vi "acquire data for calibration.vi"(0 "Connection ID":refnum<k5>, 7 "method":T2={"sampling interval"=0.1, "samples to average"=1, "data interval"=0.0, "stream data"=FALSE, "file path"=refnum, "command"={"command"=enum."Idle", "start time (ms)"=0, "Channel Indices"=[], "Scans per Sample"=1}} {"command"."Scans per Sample" min=1; "data interval" format="%.2f"; "samples to average" min=1 step=1; "sampling interval" format="%.2f"}, 9 "Reference Index":u32, 11 "Uncalibrated index":u32) -> (4 "data array":sgl[][](array[numeric]) format="%.5f", 6 "offset":sgl format="%.5f", 8 "percent CV":sgl format="%.5f")   [LabVIEW 2010]
uses:
  DataServer/Server Stats.vi
  DataServer/command.ctl
  DataServer/command cluster.ctl
  DAC apps/support/method.ctl
panel:
  in  "colors":i32[](array[numeric])=[16711680, 13311, 52224, 16777215, 16737792, 16738047, 52479, 16776960, 16711680, 13311, 52224, 16777215, 16737792, 16738047, 52479, 16776960]
  out "sample time":dbl format="%.2f"
  in  "data points to acquire":u32=1000 min=1
  out "stop":bool
  in  "State":cluster{"Monitor sample":bool, "Okay":bool}
  out "Scan rate":dbl=10.0
  out "data rate":sgl format="%.4f"
  in  "rates":T1={"Scans per Sample"=1, "samples to average"=1} {"samples to average" min=1 step=1; "Scans per Sample" min=1}
  out "sampling rate":dbl format="%.4f"
  out "chart":sgl[][](graph)
  in  "Monitoring sample":bool
  out "backlog":u32
  in  "error":errorcluster={"status"=FALSE, "code"=56, "source"="TCP Read in \u0000TCP read variable.vi->read Volts data fast.vi->Signal Monitor"}
  # "hz"
  # "s"
  # "hz"
  # "hz"
  # "s"
  # "s"
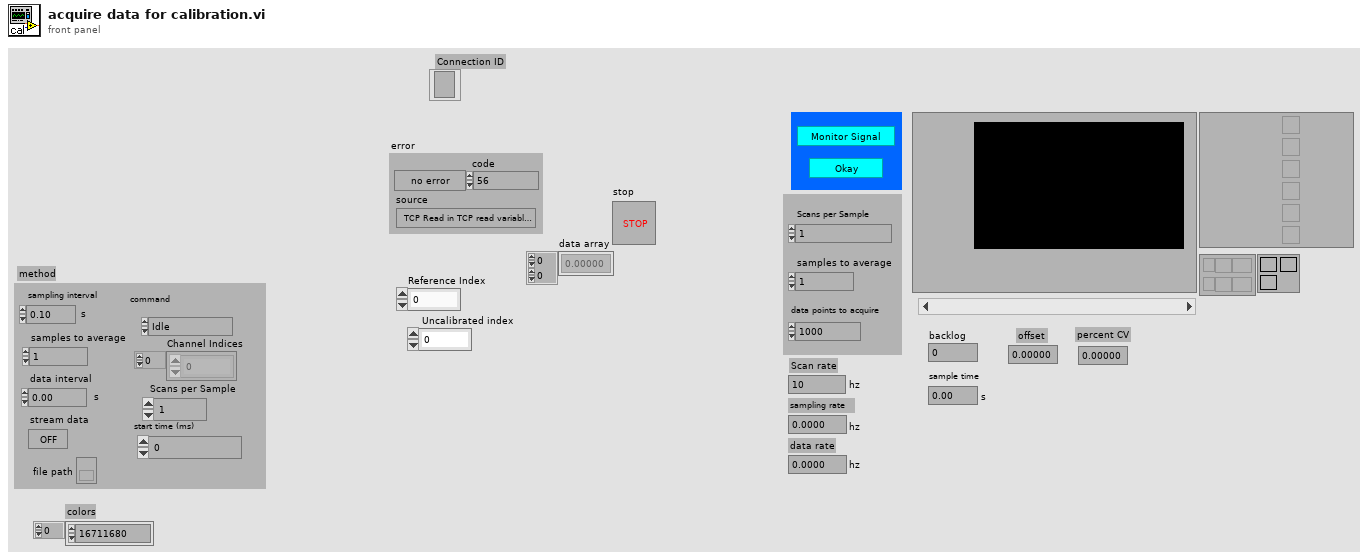
[diagram p1: front panel]
types:
  T1 = cluster{"Scans per Sample":i32, "samples to average":u32}
  T2 = typedef "method.ctl" = cluster{"sampling interval":sgl, "samples to average":u32, "data interval":sgl, "stream data":bool, "file path":refnum<file>, "command":T3}
  T3 = typedef "command cluster.ctl" = cluster{"command":T4, "start time (ms)":u32, "Channel Indices":i32[], "Scans per Sample":i32}
  T4 = typedef "command.ctl" = enum16{"Idle", "Send Data", "Send 1 Scan", "Logoff"}
  T5 = enum16{"Idle", "Send Data", "Send 1 Scan", "Logoff"}
  T6 = typedef "Server stats.ctl" = cluster{"scan rate":dbl, "# connections":i32, "channel settings":cluster{"Name":string, "upper input limits":sgl, "lower input limits":sgl, "Location":string}[]}
  T7 = cluster{"channel":string, "upper input limits":sgl, "lower input limits":sgl, "range":sgl, "polarity":enum16{"no change", "bipolar", "unipolar"}, "gain":sgl, "coupling":enum16{"no change", "DC", "AC", "ground", "internal reference"}, "input mode":enum16{"no change", "differential", "rse", "nrse"}, "scale multiplier":sgl, "scale offset":sgl}[]
  T8 = cluster{"channel":string, "upper input limits":sgl, "lower input limits":sgl, "range":sgl, "polarity":enum16{"no change", "bipolar", "unipolar"}, "gain":sgl, "coupling":enum16{"no change", "DC", "AC", "ground", "internal reference"}, "input mode":enum16{"no change", "differential", "rse", "nrse"}, "scale multiplier":sgl, "scale offset":sgl}
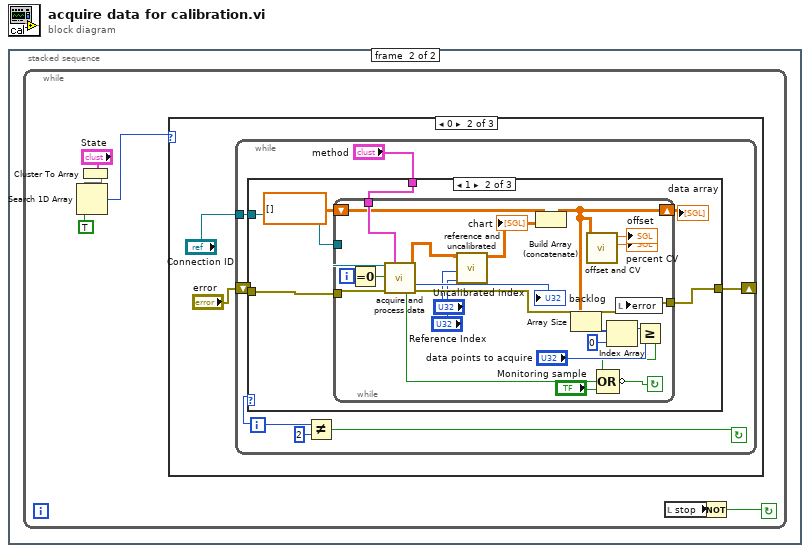
[diagram p0: block diagram]
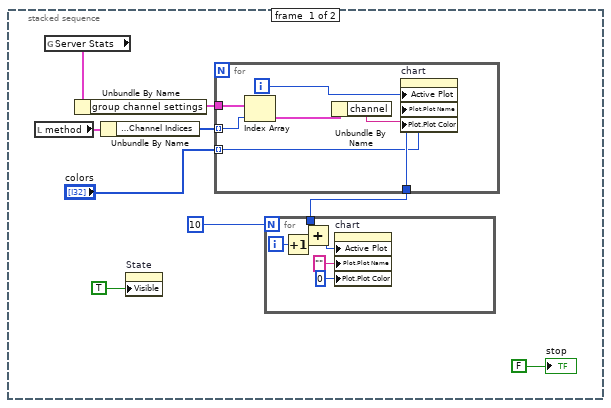
[diagram p2: hidden frame]
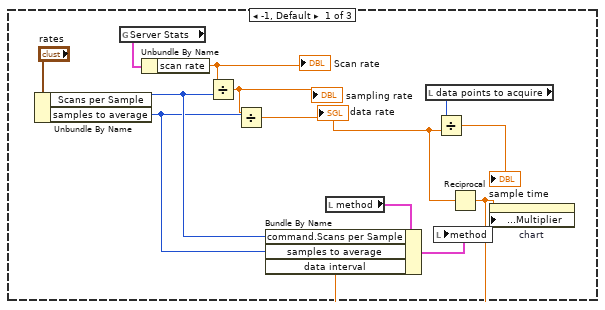
[diagram p3: hidden frame]
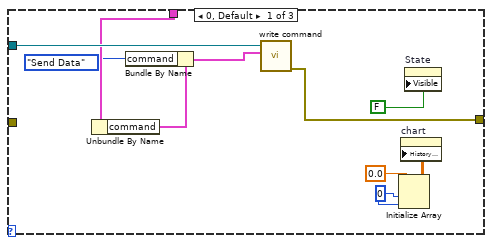
[diagram p4: hidden frame]
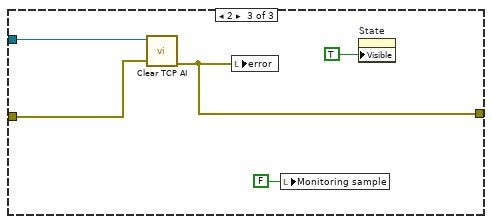
[diagram p5: hidden frame]
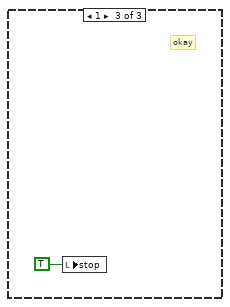
[diagram p6: hidden frame]
diagram:
  n1 = stacked-sequence {
    frame #0 {
      n2 = local read "method"() -> (w8:T2)
      n3 = global read "Server Stats.vi" "Server Stats"() -> (w1:T6)
      n4 = Unbundle By Name(w1) -> ("group channel settings"=w6:T7)
      n5 = Unbundle By Name(w8) -> ("command.Channel Indices"=w7:i32[])
      n6 = property on="State" class="Clust"("Visible"=TRUE ("Write Attribute")) -> ()  [unwired: 2 in, 2 out]
      n7 = for {
        tunnel: w7 -> [w21] mode=indexing
        tunnel: w6 -> [w20]
        tunnel: [w17] -> w4
        tunnel: "colors" -> [w16] mode=indexing
        i -> [w17]
        n8 = Index Array(array=w20, index=w21) -> (element=w19:T8)
        n9 = Unbundle By Name(w19) -> ("channel"=w18:string)
        n10 = property on="chart" class="WFChart (strict)"("Active Plot"=w17, "Plot.Plot Name"=w18, "Plot.Plot Color"=w16) -> ()  [unwired: 2 in, 2 out]
      }
      n11 = for {
        N: 10 -> [_]
        tunnel: w4 -> [w13]
        i -> [w15]
        n12 = Increment(x=w15) -> (x+1=w10:i32)
        n13 = Add(x=w13, y=w10) -> (x+y=w14:i32)
        n14 = property on="chart" class="WFChart (strict)"("Active Plot"=w14, "Plot.Plot Name"="" ("Write Attribute"), "Plot.Plot Color"=u32 0 ("Write Attribute")) -> ()  [unwired: 2 in, 2 out]
      }
      "stop" <- FALSE ("stop")
    }
    frame #1 {
      n15 = while {
        stop <- w22 continue-if-true
        n16 = Cluster To Array(cluster="State") -> (array=w27:bool[])
        n17 = Search 1D Array(1D array=w27, element=TRUE) -> (index of element=w24:i32)  [unwired: 1 in]
        n18 = case shown="0" w24 {
          frame -1, Default {
            n19 = Unbundle By Name("rates") -> ("Scans per Sample"=w34:i32, "samples to average"=w31:u32)
            n20 = global read "Server Stats.vi" "Server Stats"() -> (w28:T6)
            n21 = Unbundle By Name(w28) -> ("scan rate"=w38:dbl)
            "Scan rate" <- w38
            n22 = Divide(x=w38, y=w34) -> (x/y=w37:dbl)
            "sampling rate" <- w37
            n23 = Divide(x=w37, y=w31) -> (x/y=w30:dbl)
            "data rate" <- w30
            n24 = local read "method"() -> (w36:T2)
            n25 = local read "data points to acquire"() -> (w33:u32)
            n26 = Divide(x=w33, y=w30) -> (x/y=→"sample time":dbl)
            n27 = Reciprocal(x=w30) -> (1/x=w29:dbl)
            n28 = Bundle By Name(cluster=w36, "command.Scans per Sample"=w34, "samples to average"=w31, "data interval"=w29) -> (w35:T2)
            n29 = local write "method"(w35) -> ()
            n30 = property on="chart" class="WFChart (strict)"("X Scale.Offset and Multiplier:Multiplier"=w29) -> ()  [unwired: 2 in, 2 out]
          }
          frame 0 {
            n31 = while {
              shift-left: "error" -> [w42]
              shift-right: [w43] -> _
              tunnel: "Connection ID" -> [w47]
              i -> [w46]
              stop <- w44 continue-if-true
              n32 = case shown="1" w46 {
                tunnel: [w54 w61 w88] -> w43
                tunnel: w42 -> [_ w64 w89]
                tunnel: "method" -> [w56 w63 _]
                tunnel: w47 -> [w57 w62 w90]
                frame 0, Default {
                  w53 = 0
                  n33 = Unbundle By Name(w56) -> ("command"=w55:T3)
                  n34 = Bundle By Name(cluster=w55, "command"=T5."Send Data") -> (w58:T3)
                  n35 = call "write command.vi"("command interface"=w58, "refnum in"=w57) -> ("error out"=w54:errorcluster)  [unwired: 8 in, 1 out]
                  n36 = Initialize Array(sgl 0.0, w53, w53) -> (w51:sgl[][])
                  n37 = property on="chart" class="WFChart (strict)"("History Data"=w51) -> ()  [unwired: 2 in, 2 out]
                  n38 = property on="State" class="Clust"("Visible"=FALSE ("Write Attribute")) -> ()  [unwired: 2 in, 2 out]
                }
                frame 1 {
                  n39 = while {
                    shift-left: sgl[][] [] -> [w74]
                    shift-right: [w73] -> w60
                    tunnel: w62 -> [w80]
                    tunnel: w63 -> [w81]
                    tunnel: [w84] -> w61
                    tunnel: w64 -> [w83]
                    i -> [w66]
                    stop <- w87 continue-if-true
                    n40 = Equal To 0?(x=w66) -> (x = 0?=w65:bool)
                    n41 = call "acquire and process data.vi"("connection ID"=w80, "Reset"=w65, "error in"=w83, "method"=w81) -> ("data out"=w68:sgl[][], "backlog"=→"backlog":u32, "Status"=w82:bool, "error out"=w84:errorcluster)  [unwired: 4 in, 4 out]
                    n42 = call "reference and uncalibrated.vi"("Reference Index"="Reference Index", "uncalibrated index"="Uncalibrated index", "scaled data"=w68) -> ("reference and volts"=w67:sgl[][])  [unwired: 4 in]
                    "chart" <- w67
                    n43 = Build Array (concatenate)(w74, w67) -> (w73:sgl[][])
                    n44 = Array Size(array=w73) -> (size(s)=w79:i32[])
                    n45 = call "offset and CV.vi"("volts"=w73) -> ("percent CV"=→"percent CV":sgl, "mean"=→"offset":sgl)  [unwired: 9 in]
                    n46 = Index Array(array=w79, index=0 ("Index")) -> (element=w77:i32)
                    n47 = local write "error"(w84) -> ()
                    n48 = Greater Or Equal?(x=w77, y="data points to acquire") -> (x >= y?=w75:bool)
                    n49 = Compound Arithmetic op=OR(w75, w82, "Monitoring sample") -> (invert w87:bool)
                  }
                  "data array" <- w60
                }
                frame 2 {
                  n50 = call "Clear TCP AI.vi"("error in (no error)"=w89, "Connection ID in"=w90) -> ("error out"=w88:errorcluster)  [unwired: 8 in, 1 out]
                  n51 = local write "error"(w88) -> ()
                  n52 = local write "Monitoring sample"(FALSE ("Monitoring sample")) -> ()
                  n53 = property on="State" class="Clust"("Visible"=TRUE ("Write Attribute")) -> ()  [unwired: 2 in, 2 out]
                }
              }
              n54 = Not Equal?(x=w46, y=2) -> (x != y?=w44:bool)
            }
          }
          frame 1 {
            # "okay"
            n55 = local write "stop"(TRUE ("stop")) -> ()
          }
        }
        n56 = local read "stop"() -> (w23:bool)
        n57 = Not(x=w23) -> (.not. x?=w22:bool)
      }
    }
  }
